vi "HEWH Check Test End Time.vi"(8 "Error In":errorcluster, 9 "Do NOT Check Timer":bool, 10 "Test End Time (Sec)":dbl, 11 "A Timer":dbl) -> (0 "Error Out":errorcluster, 1 "Seconds Remaining":dbl, 2 "Test Complete":bool, 3 "Disable Station":bool)   [LabVIEW 2016]
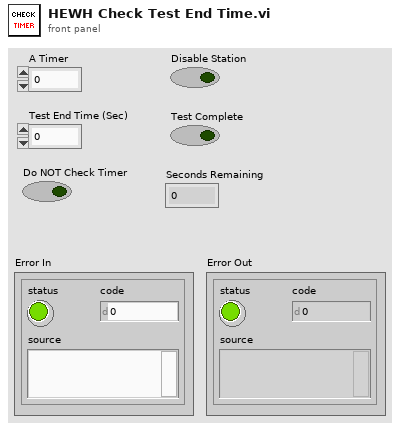
[diagram p1: front panel]
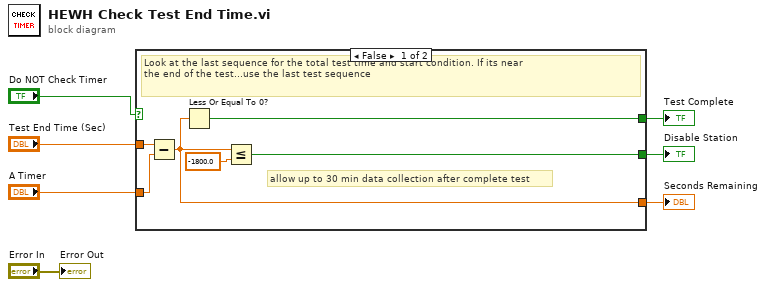
[diagram p0: block diagram]
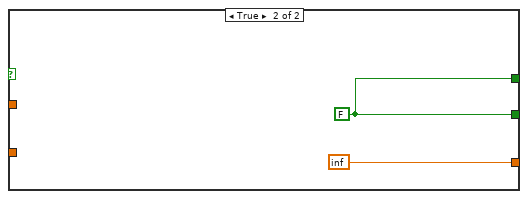
[diagram p2: hidden frame]
diagram:
  n1 = case shown="False" "Do NOT Check Timer" {
    tunnel: [w11 w14] -> w6
    tunnel: "Test End Time (Sec)" -> [w13 _]
    tunnel: "A Timer" -> [w12 _]
    tunnel: [w10 inf] -> w3
    tunnel: [w8 w14] -> w7
    frame False {
      # "allow up to 30 min data collection after complete test"
      # "Look at the last sequence for the total test time and start condition. If its near \nthe end of the test...use the last test sequence"
      n2 = Subtract(x=w13, y=w12) -> (x-y=w10:dbl)
      n3 = Less Or Equal To 0?(x=w10) -> (x <= 0?=w11:bool)
      n4 = Less Or Equal?(x=w10, y=-1800.0) -> (x <= y?=w8:bool)
    }
    frame True {
      w14 = FALSE
    }
  }
  "Disable Station" <- w7
  "Test Complete" <- w6
  "Seconds Remaining" <- w3
  "Error Out" <- "Error In"
